vi "ExportConfigurationToFile.vi"(2 "error in (no error)":errorcluster, 3 "Absolute Path of Configuration File(.zip) to Export":path, 4 "VISA resource name":refnum<visa-resource-name>) -> (0 "error out":errorcluster, 1 "VISA resource name out":refnum<visa-resource-name>)   [LabVIEW 2020, in "Active Technologies AWG3000.lvlib"]
uses:
  Active Technologies AWG3000.lvlib
panel:
  # "Note: for the drive C is allowed export a configuration only to the default folder or to its subdirectories. \nNo limitation for the other drivers.\nTo know the default folder, run GetDefaultDriveCFolder.vi."
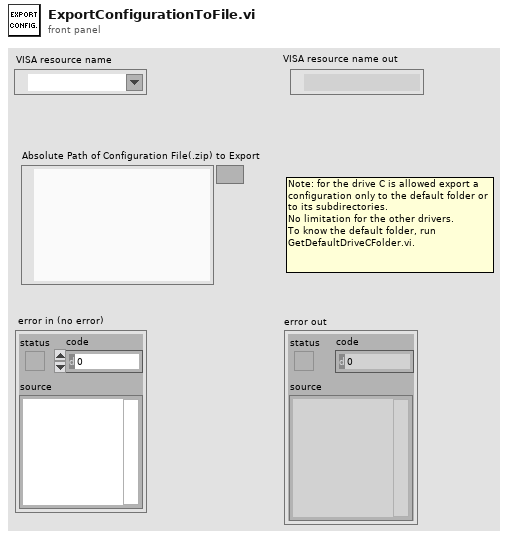
[diagram p1: front panel]
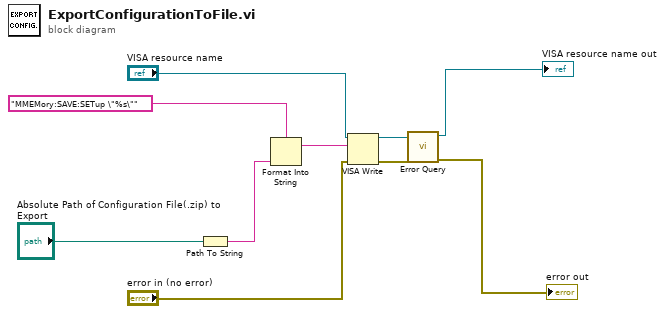
[diagram p0: block diagram]
diagram:
  n1 = Path To String(path="Absolute Path of Configuration File(.zip) to Export") -> (string=w1:string)
  n2 = Format Into String(format string="MMEMory:SAVE:SETup \"%s\"" ("write buffer"), w1) -> (resulting string=w7:string)  [unwired: 2 in, 1 out]
  n3 = VISA Write(VISA resource name="VISA resource name", write buffer=w7, error in (no error)="error in (no error)") -> (VISA resource name out=w6:refnum<visa-resource-name>, error out=w5:errorcluster)  [unwired: 1 out]
  n4 = call "Error Query.vi"("error in (no error)"=w5, "VISA resource name"=w6) -> ("error out"=→"error out":errorcluster, "VISA resource name out"=→"VISA resource name out":refnum<visa-resource-name>)  [unwired: 6 in, 2 out]
